vi "score generator.vi"(1 "Minimum":dbl=20.0, 2 "Maximum":dbl=80.0) -> (0 "score":dbl)   [LabVIEW 2014]
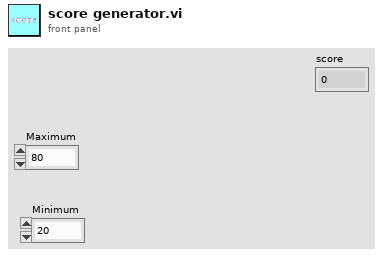
[diagram p1: front panel]
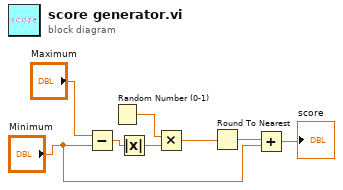
[diagram p0: block diagram]
diagram:
  n1 = Subtract(x="Maximum", y="Minimum") -> (x-y=w6:dbl)
  n2 = Random Number (0-1)() -> (number: 0 to 1=w7:dbl)
  n3 = Absolute Value(x=w6) -> (abs(x)=w4:dbl)
  n4 = Multiply(x=w7, y=w4) -> (x*y=w5:dbl)
  n5 = Round To Nearest(number=w5) -> (nearest integer value=w3:dbl)
  n6 = Add(x=w3, y="Minimum") -> (x+y=→"score":dbl)
